vi "Add Child Strings.vi"(8 "error in":errorcluster, 10 "Group_Based_Items":string[](array[string]), 11 "Report Viewer in":refnum<class "Report Viewer.lvclass">) -> (0 "error out":errorcluster, 3 "Report Viewer out":refnum<class "Report Viewer.lvclass">)   [LabVIEW 2019, in "Report Viewer.lvlib" / "Report Viewer.lvclass"]
uses:
  Library/Report Viewer.lvclass
  Library/Report Viewer.lvclass/Report Viewer.ctl
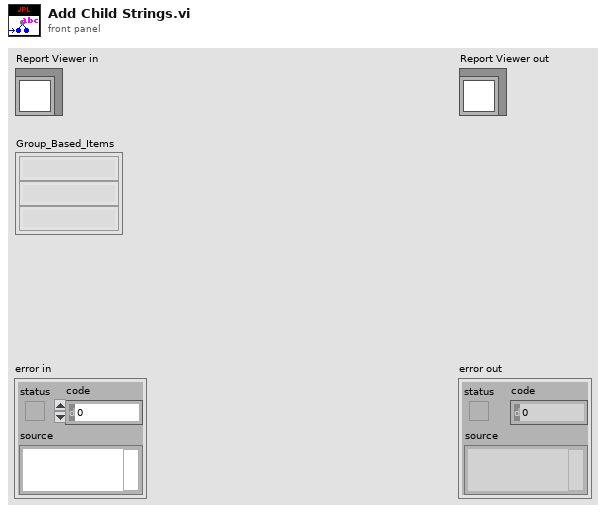
[diagram p1: front panel]
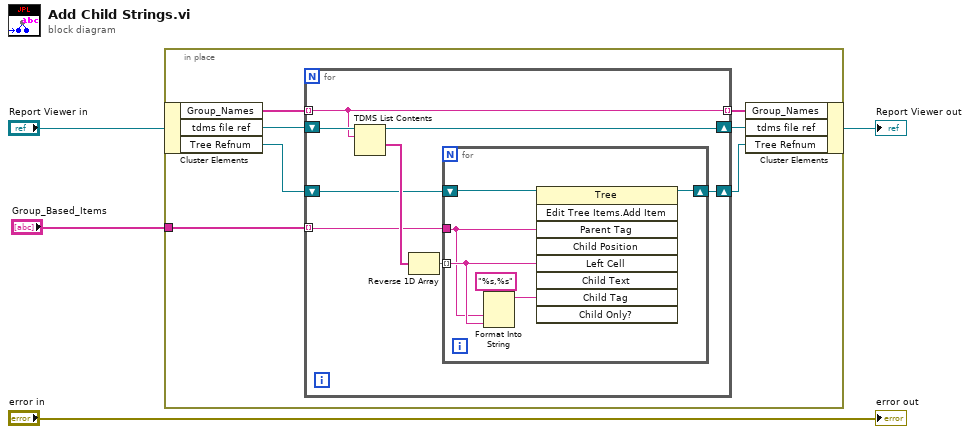
[diagram p0: block diagram]
diagram:
  n1 = in-place {
    in-place-border: "Group_Based_Items" -> [w5]
    n2 = in-place-cluster #1("Report Viewer in") -> ("Group_Names"=w11:string[], "tdms file ref"=w10:refnum<k34>, "Tree Refnum"=w7:refnum<vi>)
    n3 = for {
      tunnel: w11 -> [w12] mode=indexing
      shift-right: [w18] -> w9
      shift-left: w10 -> [w19]
      tunnel: [w12] -> w8 mode=indexing
      shift-right: [w15] -> w6
      shift-left: w7 -> [w16]
      tunnel: w5 -> [w13] mode=indexing
      n4 = TDMS List Contents(6:w12, 7:w19) -> (1:w17:string[], 3:w18:refnum<k34>)  [unwired: 1 in, 2 out]
      n5 = Reverse 1D Array(array=w17) -> (reversed array=w14:string[])
      n6 = for {
        tunnel: w14 -> [w21] mode=indexing
        tunnel: w13 -> [w20]
        shift-right: [w24] -> w15
        shift-left: w16 -> [w25]
        n7 = Format Into String(format string="%s,%s", w20, w21) -> (resulting string=w23:string)  [unwired: 2 in, 1 out]
        n8 = invoke on="Invoke Node" class="Tree" method="Edit Tree Items.Add Item"(reference=w25, "Parent Tag"=w20, "Left Cell"=w21, "Child Tag"=w23) -> (reference out=w24:refnum<vi>)  [unwired: 5 in, 8 out]
      }
    }
    n9 = in-place-cluster #1("Group_Names"=w8, "tdms file ref"=w9, "Tree Refnum"=w6) -> (→"Report Viewer out":refnum<class "Report Viewer.lvclass">)
  }
  "error out" <- "error in"
